vi "DNN Detection Model.vi"() -> ()   [LabVIEW 2020, in "examples.lvlib"]
uses:
  examples.lvlib
  feature_detection/DNN Detection Model/Detection.ctl
  feature_detection/DNN Detection Model/Rectangle Corners.ctl
  common/Image Point (Integer).ctl
  <vilib>/Utility/sysdir.llb/System Directory Type.ctl
  feature_detection/DNN Detection Model/Model Parameters.ctl
  common/Image Size (Integer).ctl
  common/Object Point (Float).ctl
  feature_detection/DNN Detection Model/DNN Detection Model.lvclass/DNN Detection Model.ctl
  image/ARGB Colour.ctl
  image/New Image (ARGB Preallocated).vi
  image/Read Image File (ARGB).vi
  feature_detection/DNN Detection Model/Detect (ARGB).vi
  image/Draw Rectangle (ARGB).vi
  image/Draw Text (ARGB).vi
  image/Draw Image to Picture (ARGB).vi
  image/New Image (ARGB Preallocated).vi/3321fa97-f432-4e1e-8db9-a0df79aed21b.vi
  image/ARGB Colour to U32 Pixel Value.vi
  image/Read Image File (ARGB).vi/2358f293-6357-4b7a-bec3-c4e4d03be6e5.vi
  feature_detection/DNN Detection Model/Detect (ARGB).vi/e837249a-f575-44a9-ab73-66ed6d7d79a4.vi
  image/Draw Rectangle (ARGB).vi/7e6fb015-3761-4366-a0a7-e436eb229083.vi
  image/Draw Text (ARGB).vi/0015c4fc-6a12-4f82-815b-6c2f827f408b.vi
  image/Draw Image to Picture (ARGB).vi/8cd07b1b-062e-4fe4-9e87-2eb3dc89fe0e.vi
  <vilib>/Utility/error.llb/Error Cluster From Error Code.vi
  feature_detection/DNN Detection Model/Create (Darknet).vi
  <vilib>/Utility/file.llb/Read Delimited Spreadsheet (string).vi
  feature_detection/DNN Detection Model/DNN Detection Model.lvclass
  common/common.lvlib
  image/image.lvlib
panel:
  out "Picture":picture
  out "error out":errorcluster
  out "Detections":T1[](array[typedef])
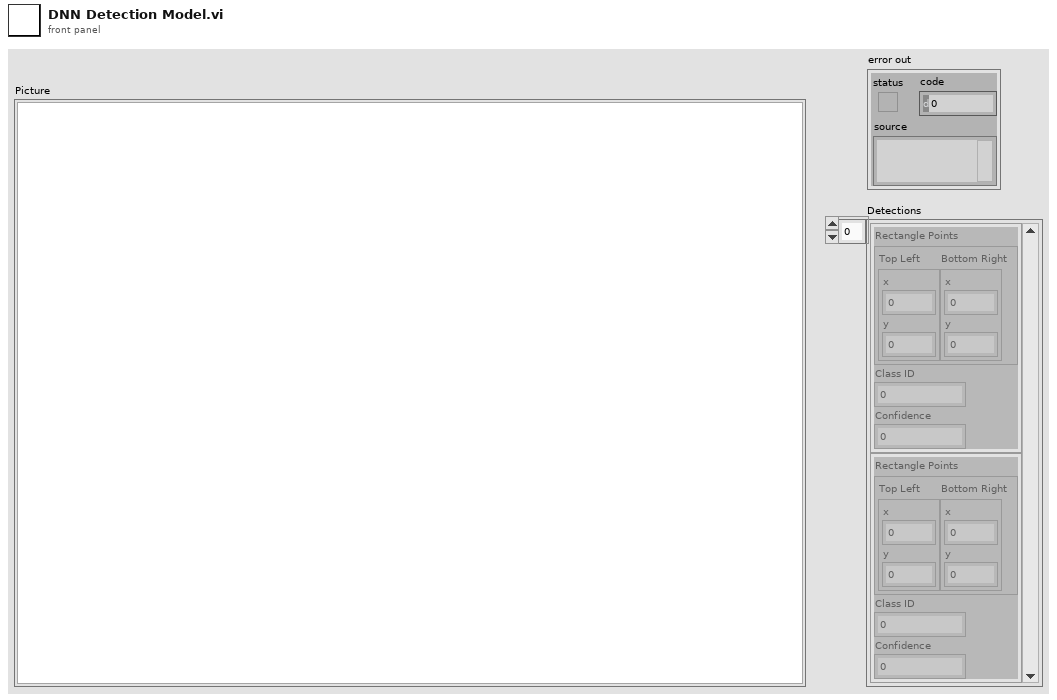
[diagram p1: front panel]
types:
  T1 = typedef "feature_detection.lvlib/DNN Detection Model.lvclass/Detection.ctl" = cluster{"Rectangle Points":T2, "Class ID":i32, "Confidence":sgl}
  T2 = typedef "feature_detection.lvlib/DNN Detection Model.lvclass/Rectangle Corners.ctl" = cluster{"Top Left":T3, "Bottom Right":T3}
  T3 = typedef "common.lvlib/Image Point (Integer).ctl" = cluster{"x":i32, "y":i32}
  T4 = typedef "feature_detection.lvlib/DNN Detection Model.lvclass/Model Parameters.ctl" = cluster{"Image Size":T5, "Mean":T6, "Scale":dbl, "Expects RGB Channel Order":bool, "Crop":bool}
  T5 = typedef "common.lvlib/Image Size (Integer).ctl" = cluster{"Width":u16, "Height":u16}
  T6 = typedef "common.lvlib/Object Point (Float).ctl" = cluster{"x":dbl, "y":dbl, "z":dbl}
  T7 = typedef "System Directory Type.ctl" = i32
  T8 = typedef "image.lvlib/ARGB Image.ctl" = refnum<data-value>
  T9 = typedef "image.lvlib/ARGB Colour.ctl" = cluster{"Alpha":u8, "RGB":u32}
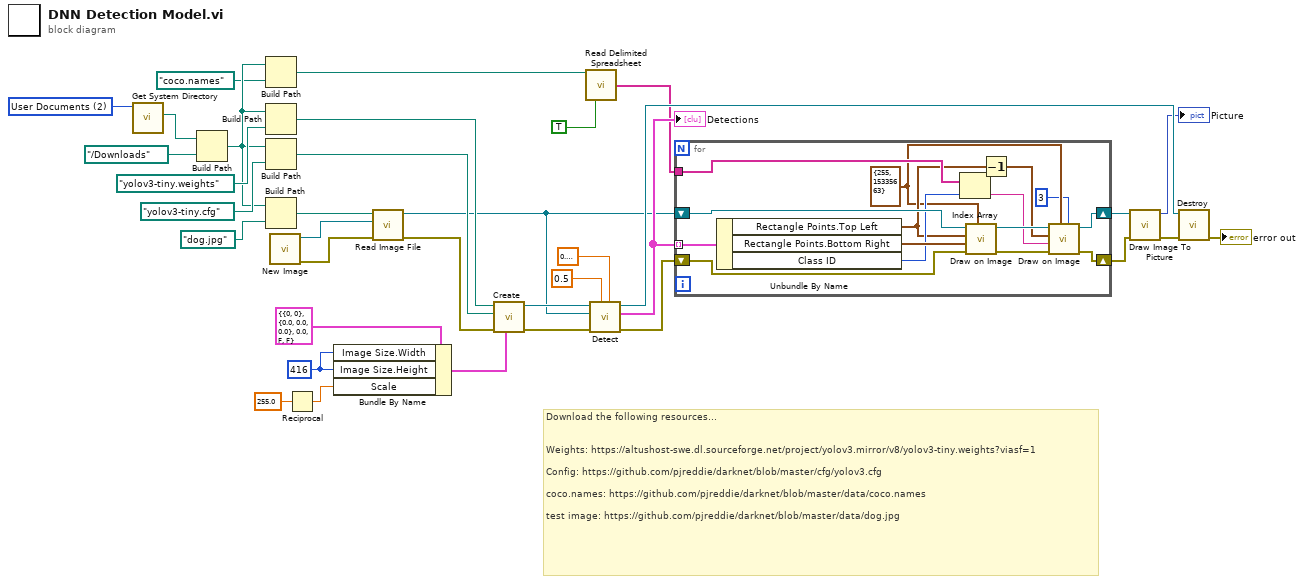
[diagram p0: block diagram]
diagram:
  w16 = u16 416 ("Image Size.Width")
  w33 = T7 2 items=["User Home"=0, "User Desktop"=1, "User Documents"=2, "User Application Data"=3, "User Preferences"=4, "User Temporary"=5, "Public Documents"=6, "Public Application Data"=7, "Public Preferences"=8, "Public Cache"=13, "System Core Libraries"=9, "System Installed Libraries"=10, "Application Files"=11, "Boot Volume Root"=12] ("system directory type")
  # "Download the following resources...\n\n\nWeights: https://altushost-swe.dl.sourceforge.net/project/yolov3.mirror/v8/yolov3-tiny.weights?viasf=1\n\nConfig: https://github.com/pjreddie/darknet/blob/master/cfg/yolov3.cfg\n\ncoco.names: https://github.com/pjreddie/darknet/blob/master/data/coco.names\n\ntest image: https://github.com/pjreddie/darknet/blob/master/data/dog.jpg"
  n1 = call <vilib>:"Get System Directory.vi"("system directory type"=w33) -> ("system directory"=w29:path)  [unwired: 10 in]
  n2 = Build Path(base path=w29, name or relative path=path "../Downloads") -> (appended path=w12:path)
  n3 = Build Path(base path=w12, name or relative path=path "coco.names") -> (appended path=w9:path)
  n4 = Build Path(base path=w12, name or relative path=path "yolov3-tiny.weights") -> (appended path=w31:path)
  n5 = Build Path(base path=w12, name or relative path=path "yolov3-tiny.cfg") -> (appended path=w27:path)
  n6 = Build Path(base path=w12, name or relative path=path "dog.jpg") -> (appended path=w23:path)
  n7 = call-poly "New Image.vi"() -> ("error out"=w21:errorcluster, "ARGB Image"=w26:T8)  [unwired: 10 in]
  n8 = Reciprocal(x=255.0) -> (1/x=w17:dbl)
  n9 = Bundle By Name(cluster=T4 {"Image Size"={"Width"=0, "Height"=0}, "Mean"={"x"=0.0, "y"=0.0, "z"=0.0}, "Scale"=0.0, "Expects RGB Channel Order"=FALSE, "Crop"=FALSE} ("Image Handling Properties"), "Image Size.Width"=w16, "Image Size.Height"=w16, "Scale"=w17) -> (w18:T4)
  n10 = call-poly "Read Image File.vi"("error in (no error)"=w21, "ARGB Image Destination in"=w26, "Filepath"=w23) -> ("error out"=w20:errorcluster, "ARGB Image Destination"=w6:T8)  [unwired: 7 in]
  n11 = call-poly "Create.vi"("Image Handling Properties"=w18, "error in (no error)"=w20, "Config (*.cfg)"=w27, "Darknet Weights (*.weights)"=w31) -> ("error out"=w22:errorcluster, "DNN Detection Model"=w34:refnum<class "DNN Detection Model.lvclass">)  [unwired: 6 in]
  n12 = call-poly <vilib>:"Read Delimited Spreadsheet.vi"("file path (dialog if empty)"=w9, "transpose? (F)"=TRUE) -> ("first row"=w5:string[])  [unwired: 8 in, 5 out]
  n13 = call-poly "Detect.vi"("Non-Maxium Suppression Threshold"=sgl 0.1, "Confidence Threshold"=sgl 0.5, "error in (no error)"=w22, "ARGB Image in"=w6, "DNN Detection Model in"=w34) -> ("error out"=w8:errorcluster, "Detections"=w7:T1[], "DNN Detection Model"=w35:refnum<class "DNN Detection Model.lvclass">)  [unwired: 4 in]
  "Detections" <- w7
  n14 = for {
    tunnel: w7 -> [w50] mode=indexing
    shift-right: [w43] -> w3
    shift-left: w8 -> [w49]
    shift-right: [w42] -> w4
    shift-left: w6 -> [w48]
    tunnel: w5 -> [w45]
    w39 = T9 {"Alpha"=255, "RGB"=15335663} ("ARGB Colour")
    n15 = Unbundle By Name(w50) -> ("Rectangle Points.Top Left"=w40:T3, "Rectangle Points.Bottom Right"=w47:T3, "Class ID"=w46:i32)
    n16 = Index Array(array=w45, index=w46) -> (element=w38:string)
    n17 = call-poly "Draw on Image.vi"("ARGB Colour"=w39, "error in (no error)"=w49, "Point B"=w47, "Point A"=w40, "ARGB Image in"=w48) -> ("error out"=w44:errorcluster, "ARGB Image"=w41:T8)  [unwired: 5 in]
    n18 = Decrement(x=w40) -> (x-1=w36:T3)
    n19 = call-poly "Draw on Image.vi"("Thickness (Default: 1)"=3, "ARGB Colour"=w39, "error in (no error)"=w44, "Text"=w38, "Origin"=w36, "ARGB Image in"=w41) -> ("error out"=w43:errorcluster, "ARGB Image"=w42:T8)  [unwired: 4 in]
  }
  n20 = call-poly "Draw Image To Picture.vi"("error in (no error)"=w3, "ARGB Image Source in"=w4) -> ("error out"=w2:errorcluster, "Picture"=→"Picture":picture)  [unwired: 8 in]
  n21 = call "Destroy.vi"("error in (no error)"=w2, "DNN Detection Model"=w35) -> ("error out"=→"error out":errorcluster)  [unwired: 9 in]
